vi "StepVals.vi"(3 "Step Values":T1, 11 "Step Array":string[](array[string])) -> (0 "SAVED":bool, 1 "output array":string[](array[string]), 2 "DONE":bool)   [LabVIEW 2023]
uses:
  StepVals.ctl
  Params.ctl
panel:
  in  "Cancel":bool
  in  "SAVE":bool
  in  "TEST":T2
  in  "PARAMS":T2
  out "number":sgl[](array[numeric])
  # "PARAMETERS"
  # "TEST"
  # "** After making changes, make sure to press the 'SAVE' button. \nIf the 'CANCEL' button is selected instead, changes will not be saved."
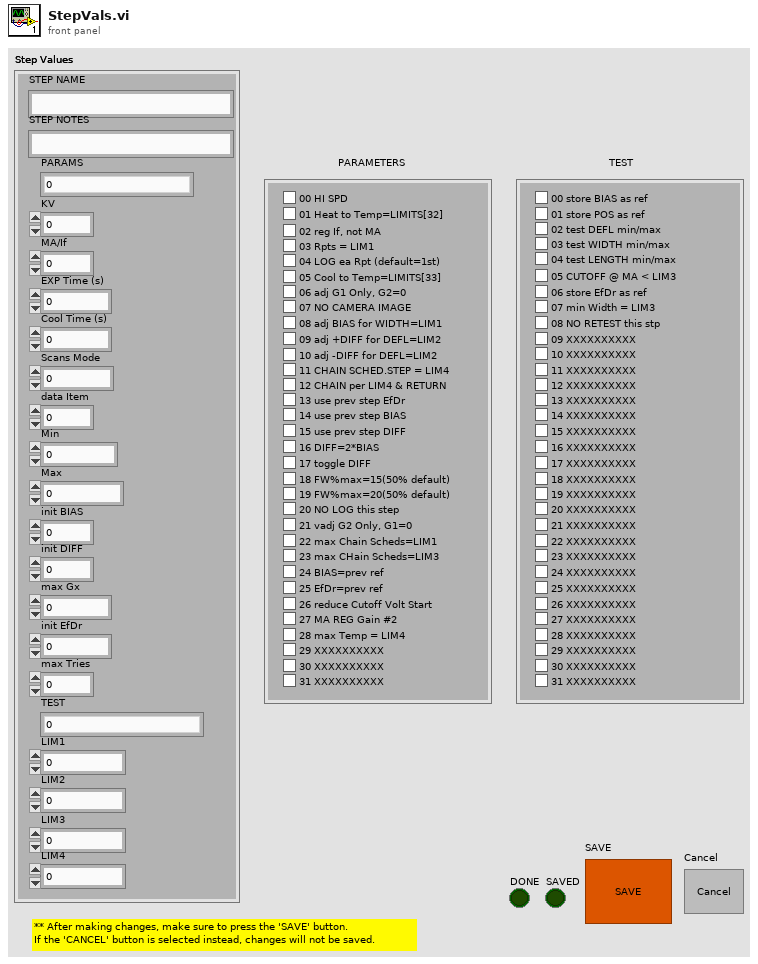
[diagram p1: front panel]
types:
  T1 = typedef "StepVals.ctl" = cluster{"STEP NAME":string, "STEP NOTES":string, "PARAMS":u32, "KV":sgl, "MA/If":sgl, "EXP Time (s)":sgl, "Cool Time (s)":sgl, "Scans Mode":sgl, "data Item":sgl, "Min":sgl, "Max":sgl, "init BIAS":sgl, "init DIFF":sgl, "max Gx":sgl, "init EfDr":sgl, "max Tries":sgl, "TEST":u32, "LIM1":sgl, "LIM2":sgl, "LIM3":sgl, "LIM4":sgl}
  T2 = typedef "Params.ctl" = cluster{"Boolean":bool, "Boolean 2":bool, "Boolean 3":bool, "Boolean 4":bool, "Boolean 5":bool, "Boolean 6":bool, "Boolean 7":bool, "Boolean 8":bool, "Boolean 9":bool, "Boolean 10":bool, "Boolean 11":bool, "Boolean 12":bool, "Boolean 13":bool, "Boolean 14":bool, "Boolean 15":bool, "Boolean 16":bool, "Boolean 17":bool, "Boolean 18":bool, "Boolean 19":bool, "Boolean 20":bool, "Boolean 21":bool, "Boolean 22":bool, "Boolean 23":bool, "Boolean 24":bool, "Boolean 25":bool, "Boolean 26":bool, "Boolean 27":bool, "Boolean 28":bool, "Boolean 29":bool, "Boolean 30":bool, "Boolean 31":bool, "Boolean 32":bool}
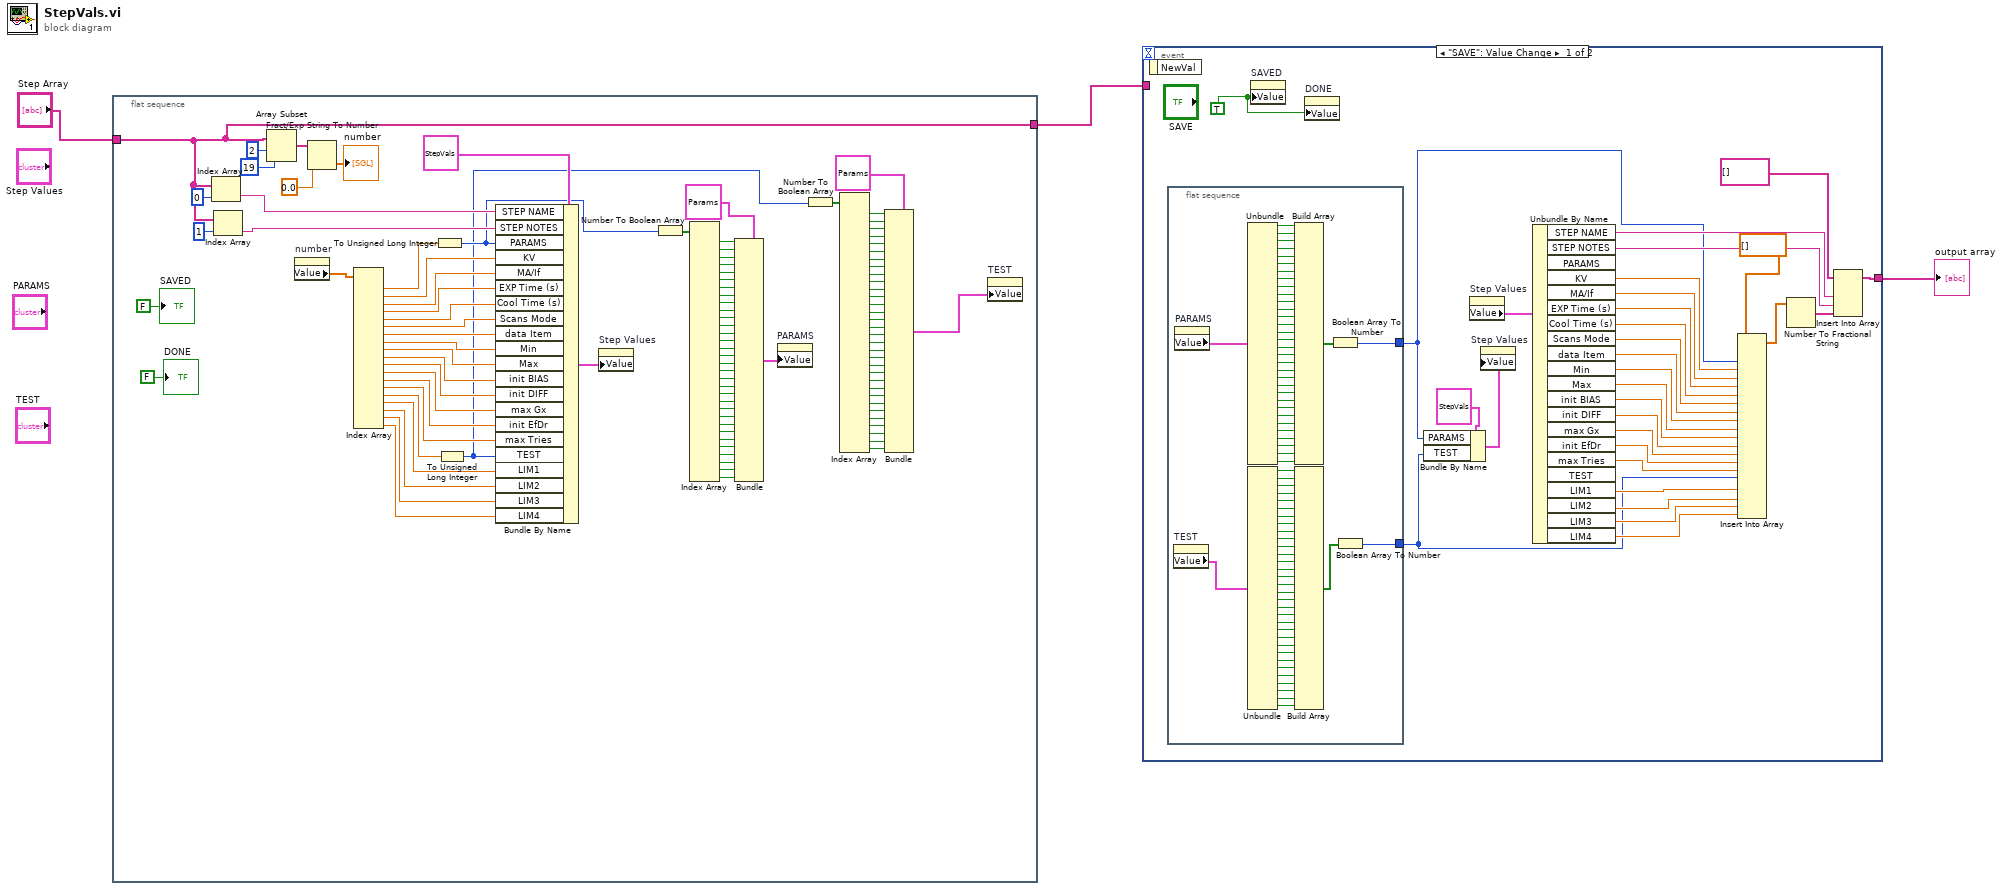
[diagram p0: block diagram]
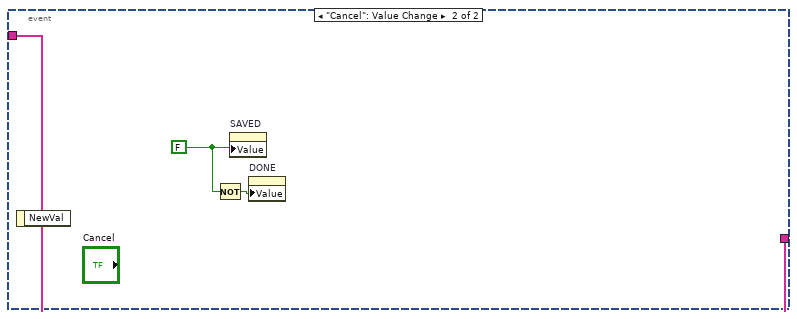
[diagram p2: hidden frame]
diagram:
  n1 = flat-sequence {
    tunnel: [w80] -> w3
    tunnel: "Step Array" -> [w80]
    frame #0 {
      n2 = Index Array(array=w80, index=0) -> (element=w88:string)
      n3 = Index Array(array=w80, index=1) -> (element=w89:string)
      n4 = Array Subset(array=w80, index=2, length=19) -> (w90:string[])
      n5 = property on="number" class="Arr (strict)"() -> ("Value"=w92:sgl[])  [unwired: 2 in, 2 out]
      n6 = Fract/Exp String To Number(string=w90, default (0 dbl)=sgl 0.0 ("default (0 DBL)")) -> (number=→"number":sgl[])  [unwired: 2 in, 1 out]
      n7 = Index Array(array=w92) -> (element #1=w11:sgl, element #2=w93:sgl, element #3=w94:sgl, element #4=w95:sgl, element #5=w96:sgl, element #6=w97:sgl, element #7=w98:sgl, element #8=w99:sgl, element #9=w100:sgl, element #10=w101:sgl, element #11=w102:sgl, element #12=w103:sgl, element #13=w104:sgl, element #14=w105:sgl, element #15=w10:sgl, element #16=w106:sgl, element #17=w107:sgl, element #18=w108:sgl, element #19=w109:sgl)  [unwired: 19 in]
      n8 = To Unsigned Long Integer(number=w11) -> (unsigned 32bit integer=w5:u32)
      n9 = To Unsigned Long Integer(number=w10) -> (unsigned 32bit integer=w4:u32)
      n10 = Bundle By Name(cluster=T1 {"STEP NAME"="WARMUP 60KV 100MA", "STEP NOTES"="PULSE KV WARMUP", "PARAMS"=130, "KV"=60.0, "MA/If"=100.0, "EXP Time (s)"=180.0, "Cool Time (s)"=300.0, "Scans Mode"=4.2, "data Item"=1.0, "Min"=1.0, "Max"=1.0, "init BIAS"=1.0, "init DIFF"=1.0, "max Gx"=1.0, "init EfDr"=85.7, "max Tries"=1.0, "TEST"=0, "LIM1"=1.0, "LIM2"=1.0, "LIM3"=1.0, "LIM4"=-1.0} ("Step Values"), "STEP NAME"=w88, "STEP NOTES"=w89, "PARAMS"=w5, "KV"=w93, "MA/If"=w94, "EXP Time (s)"=w95, "Cool Time (s)"=w96, "Scans Mode"=w97, "data Item"=w98, "Min"=w99, "Max"=w100, "init BIAS"=w101, "init DIFF"=w102, "max Gx"=w103, "init EfDr"=w104, "max Tries"=w105, "TEST"=w4, "LIM1"=w106, "LIM2"=w107, "LIM3"=w108, "LIM4"=w109) -> (w81:T1)
      n11 = property on="Step Values" class="Clust (strict)"("Value"=w81) -> ()  [unwired: 2 in, 2 out]
      n12 = Number To Boolean Array(number=w5) -> (Boolean array=w79:bool[])
      n13 = Index Array(array=w79) -> (element #1=w78:bool, element #2=w77:bool, element #3=w76:bool, element #4=w75:bool, element #5=w74:bool, element #6=w73:bool, element #7=w72:bool, element #8=w71:bool, element #9=w70:bool, element #10=w69:bool, element #11=w68:bool, element #12=w67:bool, element #13=w66:bool, element #14=w65:bool, element #15=w64:bool, element #16=w63:bool, element #17=w62:bool, element #18=w61:bool, element #19=w60:bool, element #20=w59:bool, element #21=w58:bool, element #22=w57:bool, element #23=w56:bool, element #24=w55:bool, element #25=w54:bool, element #26=w53:bool, element #27=w52:bool, element #28=w51:bool, element #29=w50:bool, element #30=w49:bool, element #31=w48:bool, element #32=w47:bool)  [unwired: 32 in]
      n14 = Bundle(cluster=T2 {"Boolean"=FALSE, "Boolean 2"=FALSE, "Boolean 3"=FALSE, "Boolean 4"=FALSE, "Boolean 5"=FALSE, "Boolean 6"=FALSE, "Boolean 7"=FALSE, "Boolean 8"=FALSE, "Boolean 9"=FALSE, "Boolean 10"=FALSE, "Boolean 11"=FALSE, "Boolean 12"=FALSE, "Boolean 13"=FALSE, "Boolean 14"=FALSE, "Boolean 15"=FALSE, "Boolean 16"=FALSE, "Boolean 17"=FALSE, "Boolean 18"=FALSE, "Boolean 19"=FALSE, "Boolean 20"=FALSE, "Boolean 21"=FALSE, "Boolean 22"=FALSE, "Boolean 23"=FALSE, "Boolean 24"=FALSE, "Boolean 25"=FALSE, "Boolean 26"=FALSE, "Boolean 27"=FALSE, "Boolean 28"=FALSE, "Boolean 29"=FALSE, "Boolean 30"=FALSE, "Boolean 31"=FALSE, "Boolean 32"=FALSE} ("PARAMS"), "Boolean"=w78, "Boolean 2"=w77, "Boolean 3"=w76, "Boolean 4"=w75, "Boolean 5"=w74, "Boolean 6"=w73, "Boolean 7"=w72, "Boolean 8"=w71, "Boolean 9"=w70, "Boolean 10"=w69, "Boolean 11"=w68, "Boolean 12"=w67, "Boolean 13"=w66, "Boolean 14"=w65, "Boolean 15"=w64, "Boolean 16"=w63, "Boolean 17"=w62, "Boolean 18"=w61, "Boolean 19"=w60, "Boolean 20"=w59, "Boolean 21"=w58, "Boolean 22"=w57, "Boolean 23"=w56, "Boolean 24"=w55, "Boolean 25"=w54, "Boolean 26"=w53, "Boolean 27"=w52, "Boolean 28"=w51, "Boolean 29"=w50, "Boolean 30"=w49, "Boolean 31"=w48, "Boolean 32"=w47) -> (w46:T2)
      n15 = property on="PARAMS" class="Clust (strict)"("Value"=w46) -> ()  [unwired: 2 in, 2 out]
      n16 = Number To Boolean Array(number=w4) -> (Boolean array=w45:bool[])
      n17 = Index Array(array=w45) -> (element #1=w44:bool, element #2=w43:bool, element #3=w42:bool, element #4=w41:bool, element #5=w40:bool, element #6=w39:bool, element #7=w38:bool, element #8=w37:bool, element #9=w36:bool, element #10=w35:bool, element #11=w34:bool, element #12=w33:bool, element #13=w32:bool, element #14=w31:bool, element #15=w30:bool, element #16=w29:bool, element #17=w28:bool, element #18=w27:bool, element #19=w26:bool, element #20=w25:bool, element #21=w24:bool, element #22=w23:bool, element #23=w22:bool, element #24=w21:bool, element #25=w20:bool, element #26=w19:bool, element #27=w18:bool, element #28=w17:bool, element #29=w16:bool, element #30=w15:bool, element #31=w14:bool, element #32=w13:bool)  [unwired: 32 in]
      n18 = Bundle(cluster=T2 {"Boolean"=FALSE, "Boolean 2"=FALSE, "Boolean 3"=FALSE, "Boolean 4"=FALSE, "Boolean 5"=FALSE, "Boolean 6"=FALSE, "Boolean 7"=FALSE, "Boolean 8"=FALSE, "Boolean 9"=FALSE, "Boolean 10"=FALSE, "Boolean 11"=FALSE, "Boolean 12"=FALSE, "Boolean 13"=FALSE, "Boolean 14"=FALSE, "Boolean 15"=FALSE, "Boolean 16"=FALSE, "Boolean 17"=FALSE, "Boolean 18"=FALSE, "Boolean 19"=FALSE, "Boolean 20"=FALSE, "Boolean 21"=FALSE, "Boolean 22"=FALSE, "Boolean 23"=FALSE, "Boolean 24"=FALSE, "Boolean 25"=FALSE, "Boolean 26"=FALSE, "Boolean 27"=FALSE, "Boolean 28"=FALSE, "Boolean 29"=FALSE, "Boolean 30"=FALSE, "Boolean 31"=FALSE, "Boolean 32"=FALSE} ("TEST"), "Boolean"=w44, "Boolean 2"=w43, "Boolean 3"=w42, "Boolean 4"=w41, "Boolean 5"=w40, "Boolean 6"=w39, "Boolean 7"=w38, "Boolean 8"=w37, "Boolean 9"=w36, "Boolean 10"=w35, "Boolean 11"=w34, "Boolean 12"=w33, "Boolean 13"=w32, "Boolean 14"=w31, "Boolean 15"=w30, "Boolean 16"=w29, "Boolean 17"=w28, "Boolean 18"=w27, "Boolean 19"=w26, "Boolean 20"=w25, "Boolean 21"=w24, "Boolean 22"=w23, "Boolean 23"=w22, "Boolean 24"=w21, "Boolean 25"=w20, "Boolean 26"=w19, "Boolean 27"=w18, "Boolean 28"=w17, "Boolean 29"=w16, "Boolean 30"=w15, "Boolean 31"=w14, "Boolean 32"=w13) -> (w12:T2)
      n19 = property on="TEST" class="Clust (strict)"("Value"=w12) -> ()  [unwired: 2 in, 2 out]
      "SAVED" <- FALSE ("SAVED")
      "DONE" <- FALSE ("DONE")
    }
  }
  n20 = event shown="[0] \"SAVE\": Value Change" {
    selector: _ -> [_ _]
    dyn-events: _ -> [_ _]
    timeout: _ -> [_ _]
    tunnel: w3 -> [_ w212]
    tunnel: [w139 w212] -> w2
    event "SAVE": Value Change {
      w138 = TRUE ("SAVED")
      n21 = event-data() -> ()  [unwired: 1 in, 1 out]
      n22 = flat-sequence {
        tunnel: [w141] -> w111
        tunnel: [w140] -> w112
        frame #0 {
          n23 = property on="TEST" class="Clust (strict)"() -> ("Value"=w143:T2)  [unwired: 2 in, 2 out]
          n24 = property on="PARAMS" class="Clust (strict)"() -> ("Value"=w145:T2)  [unwired: 2 in, 2 out]
          n25 = Unbundle(w145) -> ("Boolean"=w209:bool, "Boolean 2"=w208:bool, "Boolean 3"=w207:bool, "Boolean 4"=w206:bool, "Boolean 5"=w205:bool, "Boolean 6"=w204:bool, "Boolean 7"=w203:bool, "Boolean 8"=w202:bool, "Boolean 9"=w201:bool, "Boolean 10"=w200:bool, "Boolean 11"=w199:bool, "Boolean 12"=w198:bool, "Boolean 13"=w197:bool, "Boolean 14"=w196:bool, "Boolean 15"=w195:bool, "Boolean 16"=w194:bool, "Boolean 17"=w193:bool, "Boolean 18"=w192:bool, "Boolean 19"=w191:bool, "Boolean 20"=w190:bool, "Boolean 21"=w189:bool, "Boolean 22"=w188:bool, "Boolean 23"=w187:bool, "Boolean 24"=w186:bool, "Boolean 25"=w185:bool, "Boolean 26"=w184:bool, "Boolean 27"=w183:bool, "Boolean 28"=w182:bool, "Boolean 29"=w181:bool, "Boolean 30"=w180:bool, "Boolean 31"=w179:bool, "Boolean 32"=w178:bool)
          n26 = Unbundle(w143) -> ("Boolean"=w177:bool, "Boolean 2"=w176:bool, "Boolean 3"=w175:bool, "Boolean 4"=w174:bool, "Boolean 5"=w173:bool, "Boolean 6"=w172:bool, "Boolean 7"=w171:bool, "Boolean 8"=w170:bool, "Boolean 9"=w169:bool, "Boolean 10"=w168:bool, "Boolean 11"=w167:bool, "Boolean 12"=w166:bool, "Boolean 13"=w165:bool, "Boolean 14"=w164:bool, "Boolean 15"=w163:bool, "Boolean 16"=w162:bool, "Boolean 17"=w161:bool, "Boolean 18"=w160:bool, "Boolean 19"=w159:bool, "Boolean 20"=w158:bool, "Boolean 21"=w157:bool, "Boolean 22"=w156:bool, "Boolean 23"=w155:bool, "Boolean 24"=w154:bool, "Boolean 25"=w153:bool, "Boolean 26"=w152:bool, "Boolean 27"=w151:bool, "Boolean 28"=w150:bool, "Boolean 29"=w149:bool, "Boolean 30"=w148:bool, "Boolean 31"=w147:bool, "Boolean 32"=w146:bool)
          n27 = Build Array(w209, w208, w207, w206, w205, w204, w203, w202, w201, w200, w199, w198, w197, w196, w195, w194, w193, w192, w191, w190, w189, w188, w187, w186, w185, w184, w183, w182, w181, w180, w179, w178) -> (w144:bool[])
          n28 = Build Array(w177, w176, w175, w174, w173, w172, w171, w170, w169, w168, w167, w166, w165, w164, w163, w162, w161, w160, w159, w158, w157, w156, w155, w154, w153, w152, w151, w150, w149, w148, w147, w146) -> (w142:bool[])
          n29 = Boolean Array To Number(Boolean array=w144) -> (number=w141:u32)
          n30 = Boolean Array To Number(Boolean array=w142) -> (number=w140:u32)
        }
      }
      n31 = property on="SAVED" class="Bool (strict)"("Value"=w138) -> ()  [unwired: 2 in, 2 out]
      n32 = property on="DONE" class="Bool (strict)"("Value"=w138) -> ()  [unwired: 2 in, 2 out]
      n33 = Bundle By Name(cluster=T1 {"STEP NAME"="WARMUP 60KV 100MA", "STEP NOTES"="PULSE KV WARMUP", "PARAMS"=130, "KV"=60.0, "MA/If"=100.0, "EXP Time (s)"=180.0, "Cool Time (s)"=300.0, "Scans Mode"=4.2, "data Item"=1.0, "Min"=1.0, "Max"=1.0, "init BIAS"=1.0, "init DIFF"=1.0, "max Gx"=1.0, "init EfDr"=85.7, "max Tries"=1.0, "TEST"=0, "LIM1"=1.0, "LIM2"=1.0, "LIM3"=1.0, "LIM4"=-1.0} ("Step Values"), "PARAMS"=w111, "TEST"=w112) -> (w110:T1)
      n34 = property on="Step Values" class="Clust (strict)"() -> ("Value"=w114:T1)  [unwired: 2 in, 2 out]
      n35 = property on="Step Values" class="Clust (strict)"("Value"=w110) -> ()  [unwired: 2 in, 2 out]
      n36 = Unbundle By Name(w114) -> ("STEP NAME"=w136:string, "STEP NOTES"=w137:string, "KV"=w118:sgl, "MA/If"=w119:sgl, "EXP Time (s)"=w120:sgl, "Cool Time (s)"=w121:sgl, "Scans Mode"=w122:sgl, "data Item"=w123:sgl, "Min"=w124:sgl, "Max"=w125:sgl, "init BIAS"=w126:sgl, "init DIFF"=w127:sgl, "max Gx"=w128:sgl, "init EfDr"=w129:sgl, "max Tries"=w130:sgl, "LIM1"=w131:sgl, "LIM2"=w132:sgl, "LIM3"=w133:sgl, "LIM4"=w134:sgl)  [unwired: 2 out]
      n37 = Insert Into Array(array=dbl[] [], new element #1=w111, new element #2=w118, new element #3=w119, new element #4=w120, new element #5=w121, new element #6=w122, new element #7=w123, new element #8=w124, new element #9=w125, new element #10=w126, new element #11=w127, new element #12=w128, new element #13=w129, new element #14=w130, new element #15=w112, new element #16=w131, new element #17=w132, new element #18=w133, new element #19=w134) -> (w117:dbl[])  [unwired: 1 in]
      n38 = Number To Fractional String(number=w117) -> (F-format string=w135:string[])  [unwired: 3 in]
      n39 = Insert Into Array(array=string[] [], new element #1=w136, new element #2=w137, new element #3=w135) -> (w139:string[])  [unwired: 1 in]
    }
    event "Cancel": Value Change {
      w211 = FALSE ("SAVED")
      n40 = event-data() -> ()  [unwired: 1 in, 1 out]
      n41 = Not(x=w211) -> (.not. x?=w210:bool)
      n42 = property on="SAVED" class="Bool (strict)"("Value"=w211) -> ()  [unwired: 2 in, 2 out]
      n43 = property on="DONE" class="Bool (strict)"("Value"=w210) -> ()  [unwired: 2 in, 2 out]
    }
  }
  "output array" <- w2
